vi "S2C_SaveScript.vi"(8 "Error In":errorcluster, 11 "ScritpPathIn":path) -> (0 "Error Out":errorcluster)   [LabVIEW 2015]
doc: "Checks the script settings and saves the script to a local file."
uses:
  Globals/S2C_Globals.vi
  <vilib>/Utility/config.llb/Write Key (String).vi
  <vilib>/Utility/config.llb/NI_LVConfig.lvlib
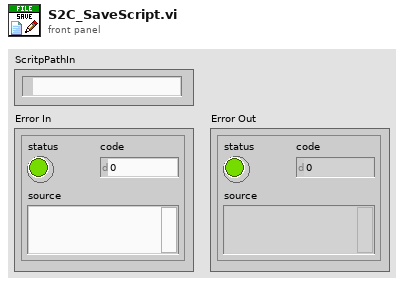
[diagram p1: front panel]
types:
  T1 = typedef "NI_LVConfig.lvlib/Config Data RefNum.ctl" = refnum<k1>
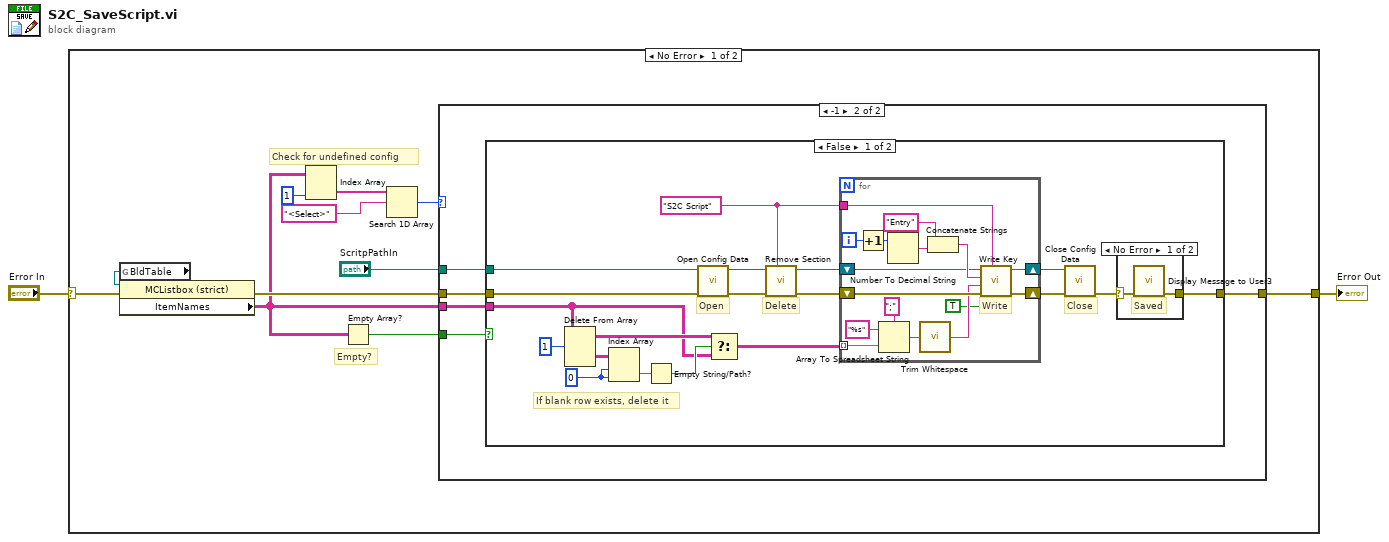
[diagram p0: block diagram]
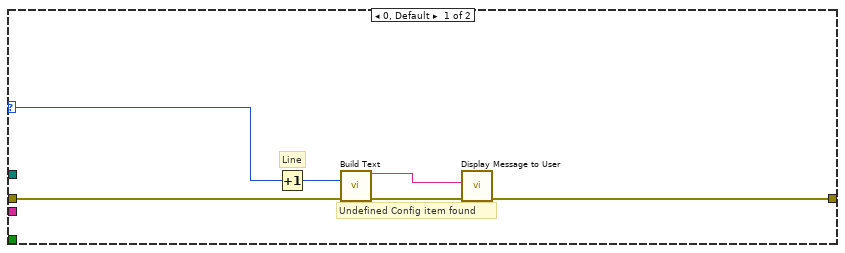
[diagram p2: hidden frame]
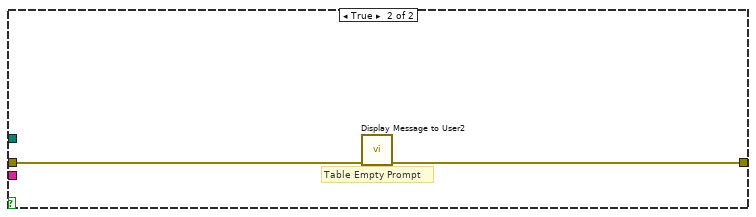
[diagram p4: hidden frame]
diagram:
  n1 = case shown="No Error" "Error In" {
    selector: "Error In" -> [w4 w65]
    tunnel: [w13 w65] -> w1
    frame No Error {
      # "Check for undefined config"
      # "Empty?"
      n2 = global read "S2C_Globals.vi" "BldTable"() -> (w11:refnum<vi>)
      n3 = property class="MCListbox (strict)"(reference=w11, error in=w4) -> (error out=w12:errorcluster, "ItemNames"=w6:string[][])  [unwired: 1 out]
      n4 = Index Array(array=w6, index (col)=1 ("disabled index (col)")) -> (element=w9:string[])  [unwired: 1 in]
      n5 = Empty Array?(array=w6) -> (empty?=w5:bool)
      n6 = Search 1D Array(1D array=w9, element="<Select>") -> (index of element=w7:i32)  [unwired: 1 in]
      n7 = case shown="-1" w7 {
        selector: w7 -> [w18 _]
        tunnel: w12 -> [w19 w24]
        tunnel: [w15 w23] -> w13
        tunnel: "ScritpPathIn" -> [_ w21]
        tunnel: w6 -> [_ w22]
        tunnel: w5 -> [_ w20]
        frame 0, Default {
          # "Line"
          # "Undefined Config item found"
          n8 = Increment(x=w18) -> (x+1=w14:i32)
          n9 = call "Build Text"("Line"=w14, "error in (no error)"=w19) -> ("Result"=w16:string, "error out"=w17:errorcluster)  [unwired: 12 in]
          n10 = call "Display Message to User"("error in (no error)"=w17, "Message"=w16) -> ("error out"=w15:errorcluster)  [unwired: 8 in, 1 out]
        }
        frame -1 {
          n11 = case shown="False" w20 {
            tunnel: w24 -> [w40 w64]
            tunnel: [w25 w63] -> w23
            tunnel: w22 -> [w28 _]
            tunnel: w21 -> [w27 _]
            frame False {
              w35 = 0 ("index (row)")
              w29 = "S2C Script"
              # "If blank row exists, delete it"
              # "Delete"
              # "Close"
              # "Open"
              n12 = Delete From Array(array=w28, length=1) -> (deleted portion=w36:string[][], array with subset deleted=w38:string[][])  [unwired: 2 in]
              n13 = Index Array(array=w36, index (row)=w35, index (col)=w35) -> (element=w34:string)
              n14 = Empty String/Path?(string/path=w34) -> (empty?=w33:bool)
              n15 = call <vilib>:"Open Config Data.vi"("error in (no error)"=w40, "configuration file path"=w27) -> ("error out"=w43:errorcluster, "refnum"=w31:T1)  [unwired: 7 in, 1 out]
              n16 = Select(t=w38, s=w33, f=w28) -> (s? t:f=w37:string[][])
              n17 = call <vilib>:"Remove Section.vi"("section"=w29, "error in (no error)"=w43, "refnum"=w31) -> ("error out"=w32:errorcluster, "refnum out"=w30:T1)  [unwired: 6 in, 1 out]
              n18 = for {
                tunnel: w37 -> [w62] mode=indexing
                shift-right: [w54] -> w42
                shift-left: w32 -> [w55]
                tunnel: w29 -> [w51]
                shift-right: [w49] -> w41
                shift-left: w30 -> [w50]
                i -> [w60]
                # "Write"
                n19 = Increment(x=w60) -> (x+1=w59:i32)
                n20 = Array To Spreadsheet String(delimiter (Tab)=";", array=w62, 3:"%s" ("format string")) -> (spreadsheet string=w53:string)
                n21 = Number To Decimal String(number=w59) -> (decimal integer string=w57:string)  [unwired: 1 in]
                n22 = call <vilib>:"Trim Whitespace.vi"("string"=w53) -> ("trimmed string"=w48:string)  [unwired: 1 in]
                n23 = Concatenate Strings("Entry" ("string"), w57) -> (w52:string)
                n24 = call-poly <vilib>:"Write Key.vi"("write raw string? (F)"=TRUE, "section"=w51, "error in (no error)"=w55, "value"=w48, "key"=w52, "refnum"=w50) -> ("error out"=w54:errorcluster, "refnum out"=w49:T1)  [unwired: 3 in, 1 out]
              }
              n25 = call <vilib>:"Close Config Data.vi"("error in (no error)"=w42, "refnum"=w41) -> ("error out"=w26:errorcluster)  [unwired: 8 in, 1 out]
              n26 = case shown="No Error" w26 {
                selector: w26 -> [w45 w46]
                tunnel: [w44 w46] -> w25
                frame No Error {
                  # "Saved"
                  n27 = call "Display Message to User3"("error in (no error)"=w45) -> ("error out"=w44:errorcluster)  [unwired: 9 in, 1 out]
                }
                frame Error {
                }
              }
            }
            frame True {
              # "Table Empty Prompt"
              n28 = call "Display Message to User2"("error in (no error)"=w64) -> ("error out"=w63:errorcluster)  [unwired: 9 in, 1 out]
            }
          }
        }
      }
    }
    frame Error {
    }
  }
  "Error Out" <- w1
